vi "Constructor.vi"(8 "error in (no error)":errorcluster, 11 "Module Settings":T1) -> (0 "error out":errorcluster, 2 "Use?":bool, 3 "Module.lvclass":refnum<class "Module.lvclass">)   [LabVIEW 2015, in "Module.lvclass"]
uses:
  Module.lvclass
  Module Settings.ctl
  Signal/Signal/Signal Settings.ctl
  Input Module/Input Module.lvclass
  Output Module/Output Module.lvclass
  Module.lvclass/Module.ctl
  Signal/Signal/Signal.lvclass
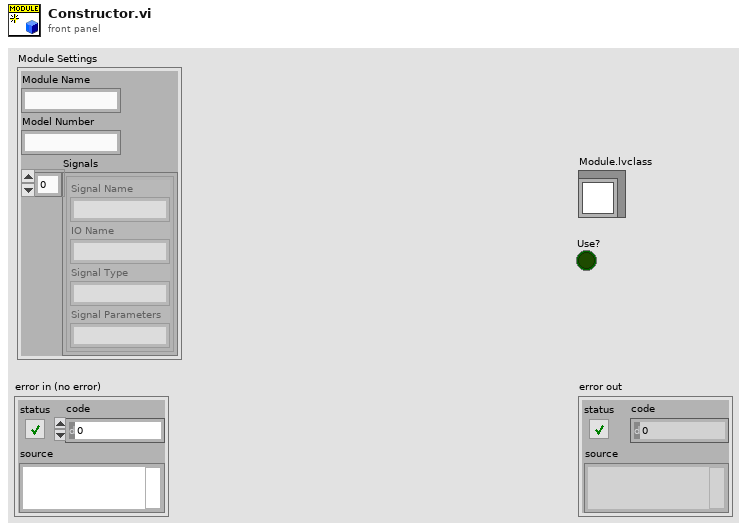
[diagram p1: front panel]
types:
  T1 = typedef "Module.lvclass/Module Settings.ctl" = cluster{"Module Name":string, "Model Number":string, "Signals":T2[]}
  T2 = typedef "Signal.lvclass/Signal Settings.ctl" = cluster{"Signal Name":string, "IO Name":string, "Signal Type":string, "Signal Parameters":string}
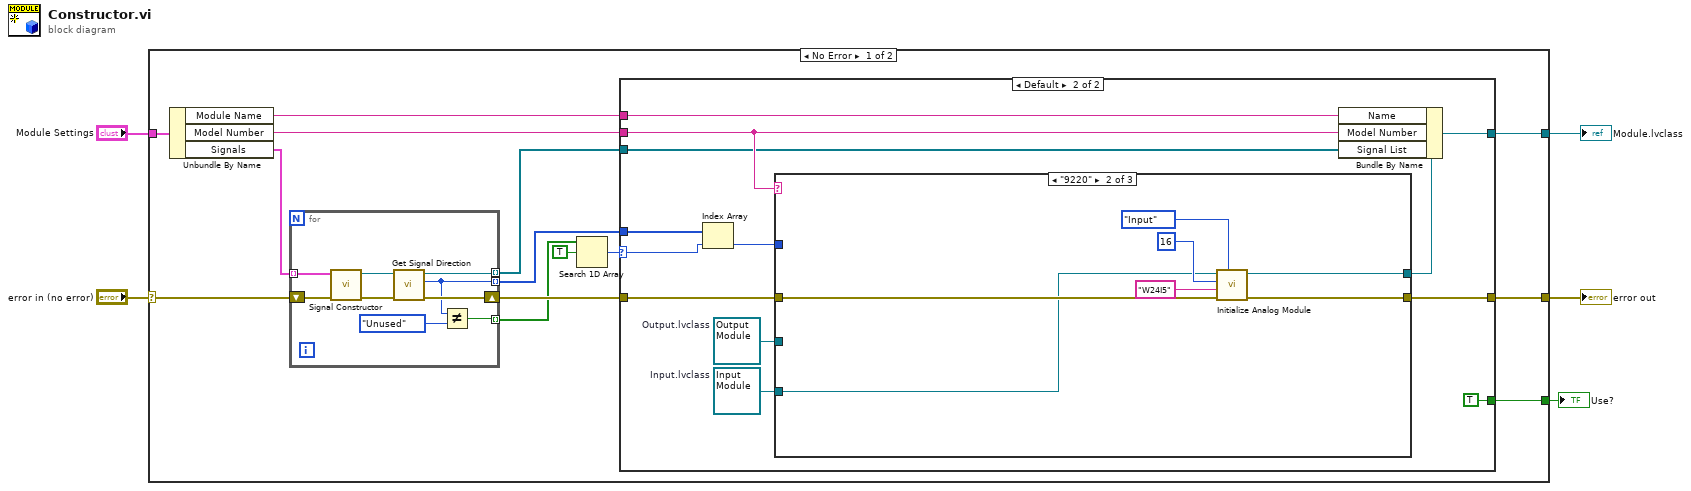
[diagram p0: block diagram]
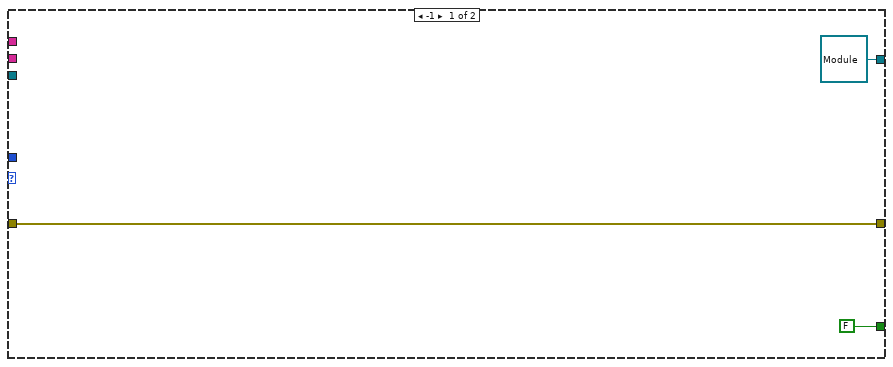
[diagram p2: hidden frame]
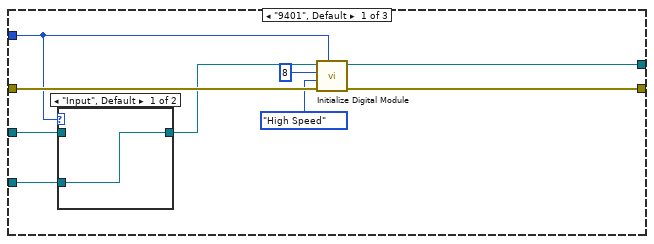
[diagram p3: hidden frame]
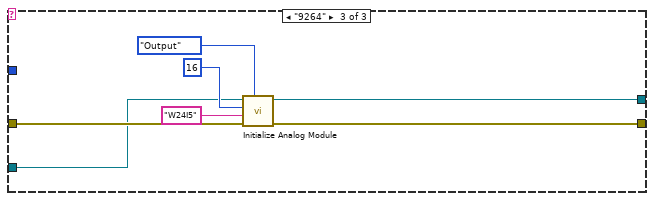
[diagram p5: hidden frame]
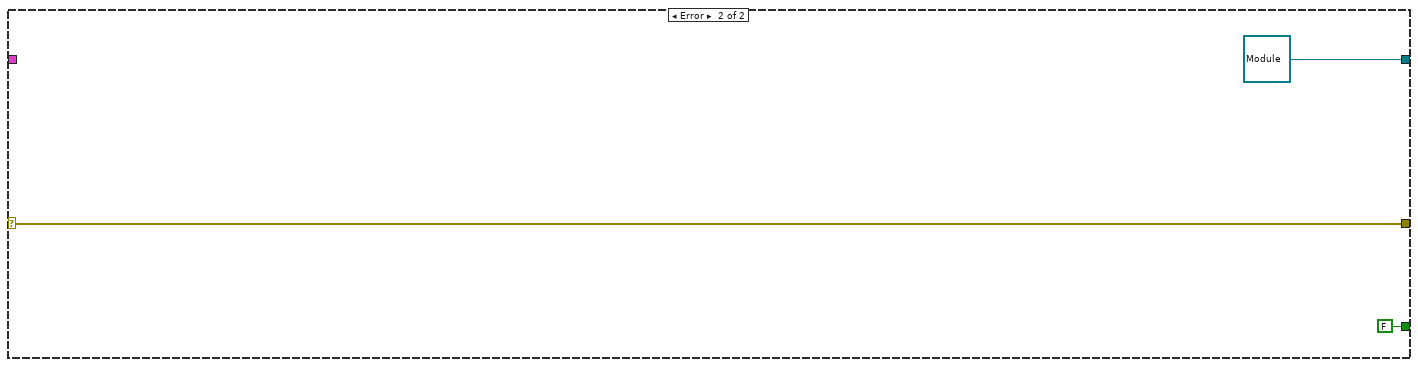
[diagram p6: hidden frame]
diagram:
  n1 = case shown="No Error" "error in (no error)" {
    selector: "error in (no error)" -> [w13 w72]
    tunnel: "Module Settings" -> [w19 _]
    tunnel: [w18 refnum<class "Module.lvclass"> refnum ("Module out")] -> w4
    tunnel: [w15 w72] -> w2
    tunnel: [w6 FALSE] -> w1
    frame No Error {
      n2 = Unbundle By Name(w19) -> ("Module Name"=w17:string, "Model Number"=w16:string, "Signals"=w14:T2[])
      n3 = for {
        tunnel: w14 -> [w69] mode=indexing
        shift-right: [w66] -> w11
        shift-left: w13 -> [w68]
        tunnel: [w64] -> w12 mode=indexing
        tunnel: [w63] -> w8 mode=indexing
        tunnel: [w61] -> w10 mode=indexing
        n4 = call "Signal Constructor.vi"("error in (no error)"=w68, "Signal Settings"=w69) -> ("error out"=w67:errorcluster, "IO Class.lvclass"=w65:refnum<class "Signal.lvclass">)  [unwired: 8 in]
        n5 = call "Get Signal Direction.vi"("error in (no error)"=w67, "IO Class in"=w65) -> ("error out"=w66:errorcluster, "Direction"=w63:enum16{"Input", "Output", "Unused"}, "IO Class out"=w64:refnum<class "Signal.lvclass">)  [unwired: 7 in]
        n6 = Not Equal?(x=w63, y=enum16{"Input", "Output", "Unused"}."Unused" ("Direction")) -> (x != y?=w61:bool)
      }
      n7 = Search 1D Array(1D array=w10, element=TRUE) -> (index of element=w7:i32)  [unwired: 1 in]
      n8 = case shown="Default" w7 {
        selector: w7 -> [_ w24]
        tunnel: [refnum<class "Module.lvclass"> refnum ("Module out") w34] -> w18
        tunnel: w17 -> [_ w33]
        tunnel: w16 -> [_ w32]
        tunnel: [w22 w31] -> w15
        tunnel: w12 -> [_ w28]
        tunnel: w11 -> [w22 w27]
        tunnel: w8 -> [_ w26]
        tunnel: [FALSE TRUE] -> w6
        frame -1 {
        }
        frame Default {
          w29 = refnum<class "Output Module.lvclass"> refnum  # Output.lvclass
          w30 = refnum<class "Input Module.lvclass"> refnum  # Input.lvclass
          n9 = Index Array(array=w26, index=w24) -> (element=w25:enum16{"Input", "Output", "Unused"})
          n10 = case shown="\"9220\"" w32 {
            tunnel: [w44 w53 w60] -> w35
            tunnel: w27 -> [w43 w48 w59]
            tunnel: [w42 w52 w58] -> w31
            tunnel: w25 -> [w39 _ _]
            tunnel: w30 -> [w37 w47 _]
            tunnel: w29 -> [w38 _ w54]
            frame "9401", Default {
              n11 = case shown="\"Input\", Default" w39 {
                tunnel: w38 -> [_ w46]
                tunnel: w37 -> [w45 _]
                tunnel: [w45 w46] -> w36
                frame "Input", Default {
                }
                frame "Output" {
                }
              }
              n12 = call "Initialize Digital Module.vi"("Direction"=w39, "error in (no error)"=w43, "Speed"=enum16{"High Speed", "Low Speed"}."High Speed", "Channels"=u8 8, "Module in"=w36) -> ("error out"=w42:errorcluster, "Module out"=w44:refnum<class "Module.lvclass">)  [unwired: 5 in]
            }
            frame "9220" {
              n13 = call "Initialize Analog Module.vi"("Direction"=enum16{"Input", "Output"}."Input", "error in (no error)"=w48, "FXP Type"="W24I5", "Channels"=u8 16, "Module in"=w47) -> ("error out"=w52:errorcluster, "Module out"=w53:refnum<class "Input Module.lvclass">)  [unwired: 5 in]
            }
            frame "9264" {
              n14 = call "Initialize Analog Module.vi"("Direction"=enum16{"Input", "Output"}."Output", "error in (no error)"=w59, "FXP Type"="W24I5", "Channels"=u8 16, "Module in"=w54) -> ("error out"=w58:errorcluster, "Module out"=w60:refnum<class "Output Module.lvclass">)  [unwired: 5 in]
            }
          }
          n15 = Bundle By Name(cluster=w35, "Name"=w33, "Model Number"=w32, "Signal List"=w28) -> (w34:refnum<class "Module.lvclass">)
        }
      }
    }
    frame Error {
    }
  }
  "Module.lvclass" <- w4
  "error out" <- w2
  "Use?" <- w1
